vi "BCtr1.vi"() -> ()   [LabVIEW 2015]
uses:
  <vilib>/Instr/_visa.llb/VISA Configure Serial Port (Instr).vi
panel:
  out "EOS":bool
  in  "StartIdx":i32
  in  "StrIn":string="M123mabcU3"
  out "Err":bool
  out "Idx":dbl
  out "error out":errorcluster
  out "Value":dbl
  out "Mode":string
  out "Modes":string[](array[string])
  out "Values":dbl[](array[numeric])
  out "Remaining":string
  out "Waveform Chart":u32(graph)
  out "Init":bool
  out "Reset":bool
  in  "Enable":bool
  in  "NB":u16[](array[numeric])
  in  "NA":u16[](array[numeric])
  in  "NC":u32 max=16777215 step=1
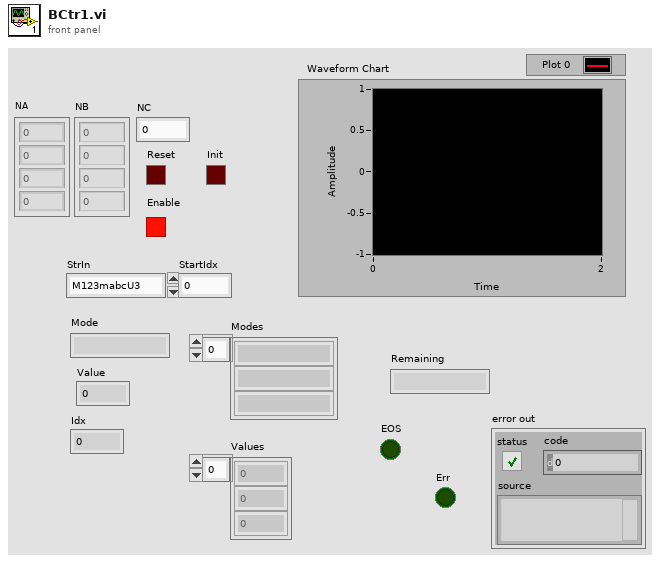
[diagram p1: front panel]
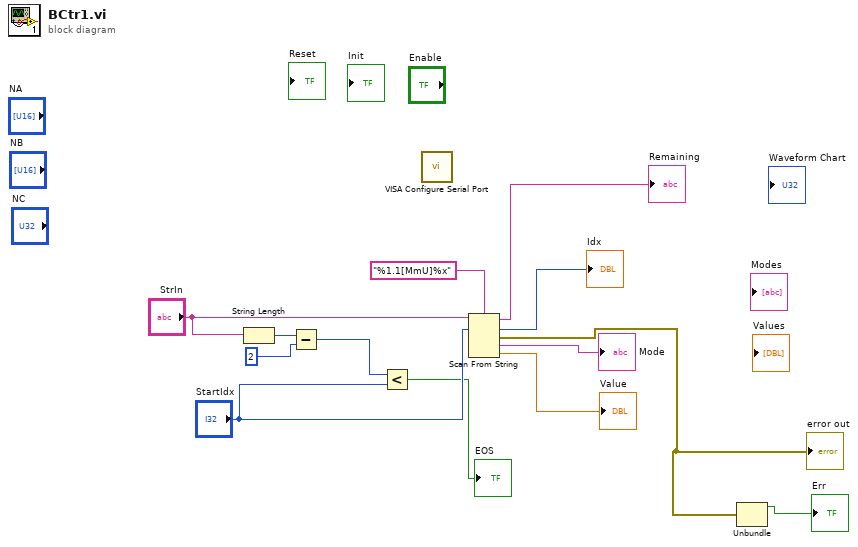
[diagram p0: block diagram]
diagram:
  n1 = String Length(string="StrIn") -> (length=w6:i32)
  n2 = Subtract(x=w6, y=2) -> (x-y=w4:i32)
  n3 = Less?(x=w4, y="StartIdx") -> (x < y?=→"EOS":bool)
  n4 = call-poly "VISA Configure Serial Port"() -> ()  [unwired: 14 in, 2 out]
  n5 = Scan From String(format string="%1.1[MmU]%x", input string="StrIn", initial scan location="StartIdx") -> (remaining string=→"Remaining":string, offset past scan=→"Idx":u32, error out=w8:errorcluster, output 1=→"Mode":string, output 2=→"Value":dbl)  [unwired: 3 in]
  "error out" <- w8
  n6 = Unbundle(w8) -> ("status"=→"Err":bool)  [unwired: 2 out]
